vi "JKI Array to Arguments.vi"(0 "Argument":string[](array[string]), 1 "Delimiter (,)":string=",") -> (4 "Arguments":string)   [LabVIEW 2017]
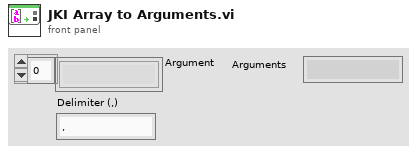
[diagram p1: front panel]
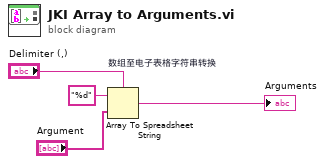
[diagram p0: block diagram]
diagram:
  n1 = Array To Spreadsheet String "数组至电子表格字符串转换"(delimiter (Tab)="Delimiter (,)", array="Argument", 3:"%d" ("格式字符串")) -> (spreadsheet string=→"Arguments":string)
